vi "LWXPS_MultipleAxesPVTParametersGet.vi"(8 "LabVIEW error IN":errorcluster, 10 "Group Name":string, 11 "XPS Reference IN":refnum<k24>) -> (0 "XPS Error String":string, 1 "Current Element Number":i32, 2 "Trajectory File Name":string, 3 "Returned error code":i32, 4 "LabVIEW error OUT":errorcluster, 5 "XPS Reference OUT":refnum<k24>)   [LabVIEW 2014]
uses:
  D:/XPSQ8_LabView_Library/Development/Source/Dll/Newport.XPS.CommandInterface.dll
  Dll/Newport.XPS.CommandInterface.dll
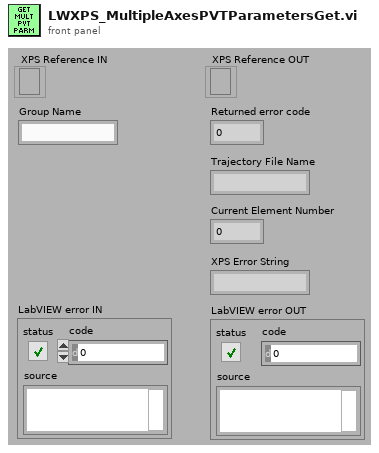
[diagram p1: front panel]
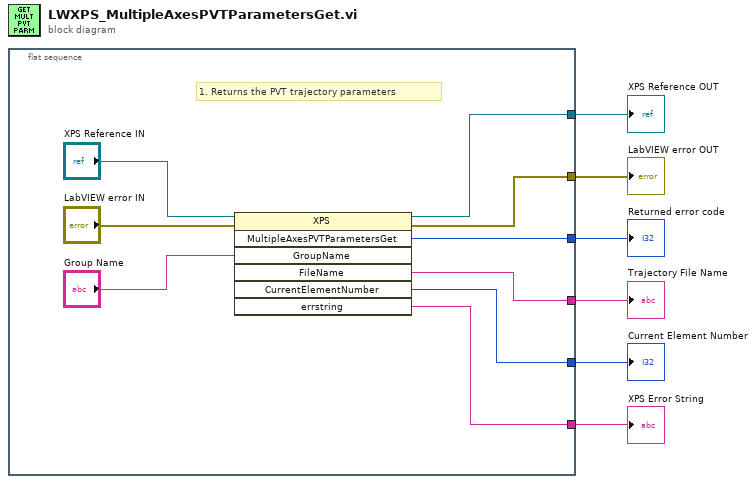
[diagram p0: block diagram]
diagram:
  n1 = flat-sequence {
    tunnel: [w13] -> w6
    tunnel: [w15] -> w5
    tunnel: [w12] -> w4
    tunnel: [w9] -> w1
    tunnel: [w8] -> w2
    tunnel: [w7] -> w3
    frame #0 {
      # "1. Returns the PVT trajectory parameters"
      n2 = invoke class="XPS" method="MultipleAxesPVTParametersGet"(reference="XPS Reference IN", error in="LabVIEW error IN", "GroupName"="Group Name") -> (reference out=w13:refnum<k24>, error out=w15:errorcluster, "MultipleAxesPVTParametersGet"=w12:i32, "FileName"=w8:string, "CurrentElementNumber"=w9:i32, "errstring"=w7:string)  [unwired: 4 in, 1 out]
    }
  }
  "XPS Reference OUT" <- w6
  "LabVIEW error OUT" <- w5
  "Returned error code" <- w4
  "XPS Error String" <- w3
  "Trajectory File Name" <- w2
  "Current Element Number" <- w1
